vi "705_ProjectA.vi"() -> ()   [LabVIEW 2015]
uses:
  <vilib>/Utility/error.llb/DialogType.ctl
  <vilib>/Platform/TimedLoop/XDataNode/timing_clust.ctl
  <vilib>/Platform/TimedLoop/XDataNode/nitl_modes.ctl
  <vilib>/Platform/TimedLoop/XDataNode/wakeup.ctl
  <vilib>/DAQmx/read.llb/DAQmx Read (Digital Bool 1Line 1Point).vi
  <vilib>/DAQmx/read.llb/DAQmx Read (Counter DBL 1Chan 1Samp).vi
  <vilib>/DAQmx/write.llb/DAQmx Write (Analog DBL 1Chan 1Samp).vi
  <vilib>/DAQmx/read.llb/DAQmx Read (Analog 1D DBL NChan 1Samp).vi
  <vilib>/DAQmx/create/channels.llb/DAQmx Create Channel (AI-Voltage-Basic).vi
  <vilib>/DAQmx/create/channels.llb/DAQmx Create Channel (AO-Voltage-Basic).vi
  <vilib>/DAQmx/create/channels.llb/DAQmx Create Channel (CI-Count Edges).vi
  <vilib>/DAQmx/create/channels.llb/DAQmx Create Channel (DI-Digital Input).vi
  Global 1.vi
  <vilib>/DAQmx/miscellaneous.llb/DAQmx Fill In Error Info.vi
  <vilib>/Analysis/3filter.llb/Butterworth Filter (DBL).vi
  <vilib>/Platform/TimedLoop/XDataNode/XDataNode.xnode
  <vilib>/Platform/TimedLoop/XDataNode/XDNodeRunTimeDep.lvlib
  <vilib>/ptbypt/NI_PtbyPt.lvlib
  <vilib>/Analysis/NI_AALBase.lvlib
panel:
  in  "stop":bool
  out "Encoder":dbl
  out "position":dbl
  out "Current Position":dbl(graph)
  in  "RESET":bool
  out "timer":dbl
  out "Motor Speed":dbl[](graph)
  out "Current Draw":dbl(graph)
  out "DAQ O/P and Motor Voltage":cluster{dbl, "Applied Motor Voltage":dbl}(graph)
  out "Motor Position 2":dbl(graph)
  out "Motor Acceleration":dbl(graph)
  in  "Tab Control":T1(tab)
  in  "Physical Channel Current":tag="Dev5/ai0"
  in  "Physical Channel Tachometer":tag="Dev5/ai0"
  in  "Physical Channel Voltage":tag="Dev5/ai0"
  in  "max moter voltage":dbl
  in  "min moter voltage":dbl
  in  "Time Period (ms)":dbl
  in  "Motor Voltage Applied":dbl(slide) min=-5.0 max=5.0 step=0.1 scale=-5.0..5.0 scale format="%#.2g"
  out "element 2":bool
  out "Motor Position":dbl
  in  "counter":tag
  in  "Lines Port0/line6":tag
  in  "Start Moving":bool
  in  "Position between gripper":dbl
  out "Position":cluster{dbl, "Position between gripper":dbl}(graph)
  in  "pVoltage Range":cluster{"output high":dbl, "output low":dbl}={"output high"=100.0, "output low"=-100.0}
  in  "pPID gains":T2={"proportional gain (Kp)"=1.0, "integral gain (Ki)"=0.01, "derivative gain (Kd)"=0.0} {"derivative gain (Kd)" format="%.3f"; "integral gain (Ki)" format="%.3f"; "proportional gain (Kp)" format="%.3f"}
  in  "Start Gripping":bool
  in  "Desired Force":dbl
  out "Force":cluster{"Desired Force":dbl, dbl}(graph)
  in  "fVoltage Range":cluster{"output high":dbl, "output low":dbl}
  in  "fPID gains":T2={"proportional gain (Kp)"=1.0, "integral gain (Ki)"=0.01, "derivative gain (Kd)"=0.0} {"derivative gain (Kd)" format="%.3f"; "integral gain (Ki)" format="%.3f"; "proportional gain (Kp)" format="%.3f"}
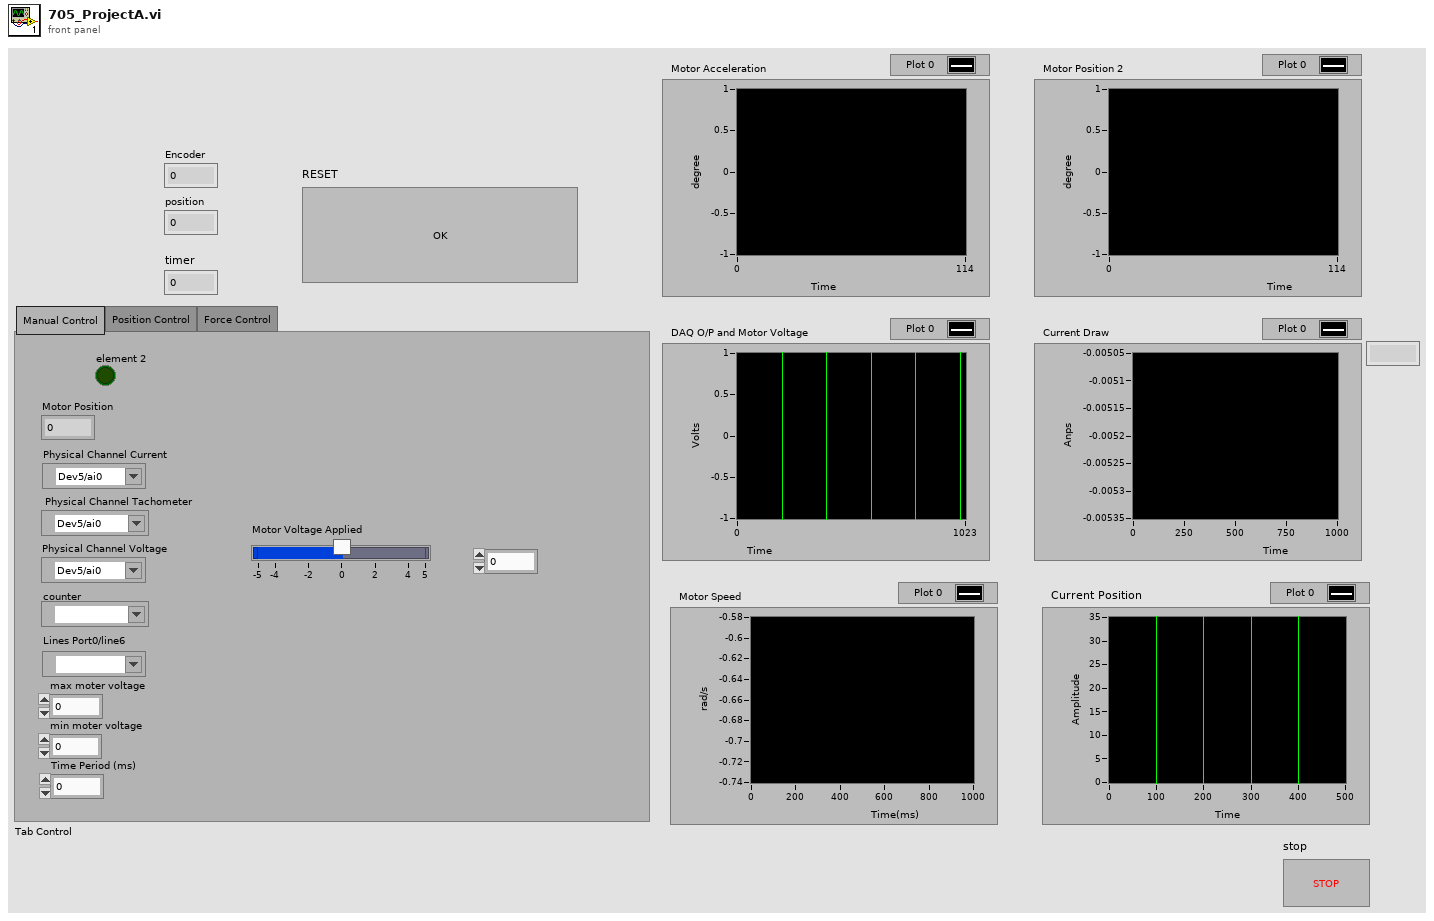
[diagram p1: front panel]
types:
  T1 = enum32{"Manual Control", "Position Control", "Force Control"}
  T2 = cluster{"proportional gain (Kp)":dbl, "integral gain (Ki)":dbl, "derivative gain (Kd)":dbl}
  T3 = typedef "DialogType.ctl" = u16
  T4 = typedef "XDNodeRunTimeDep.lvlib/timing_clust.ctl" = cluster{"Expected End [f-1]":u64, "Actual End [f-1]":u64, "Finished Late? [f-1]":bool, "Expected End [i-1]":u64, "Actual End [i-1]":u64, "Finished Late? [i-1]":bool, "Expected Start [i]":u64, "Actual Start [i]":u64, "Expected Start [f]":u64, "Actual Start [f]":u64, "Source Name":string, "Structure Name":string, "Period":i64, "Deadline":i64, "Offset":i64, "Start":i64, "Priority":i32, "Timeout":i32, "Mode":T5, "Wakeup Reason":T6, "Error":errorcluster, "Source Type":string, "Secondary Source Type":string, "Global End Time":u64, "Global Start Time":u64, "Frame Duration":u64, "Iteration Duration":u64, "Assigned CPU":i32, "I/O Scan Engine Mode":u32}
  T5 = typedef "XDNodeRunTimeDep.lvlib/nitl_modes.ctl" = enum32{"No Change", "Process missed periods, maintain original phase", "Discard missed periods, maintain original phase", "Process missed periods, ignore original phase", "Discard missed periods, ignore original phase"}
  T6 = typedef "XDNodeRunTimeDep.lvlib/wakeup.ctl" = enum32{"Normal", "Aborted", "Asynchronous wakeup", "Timing source error", "Timed loop error", "Timeout"}
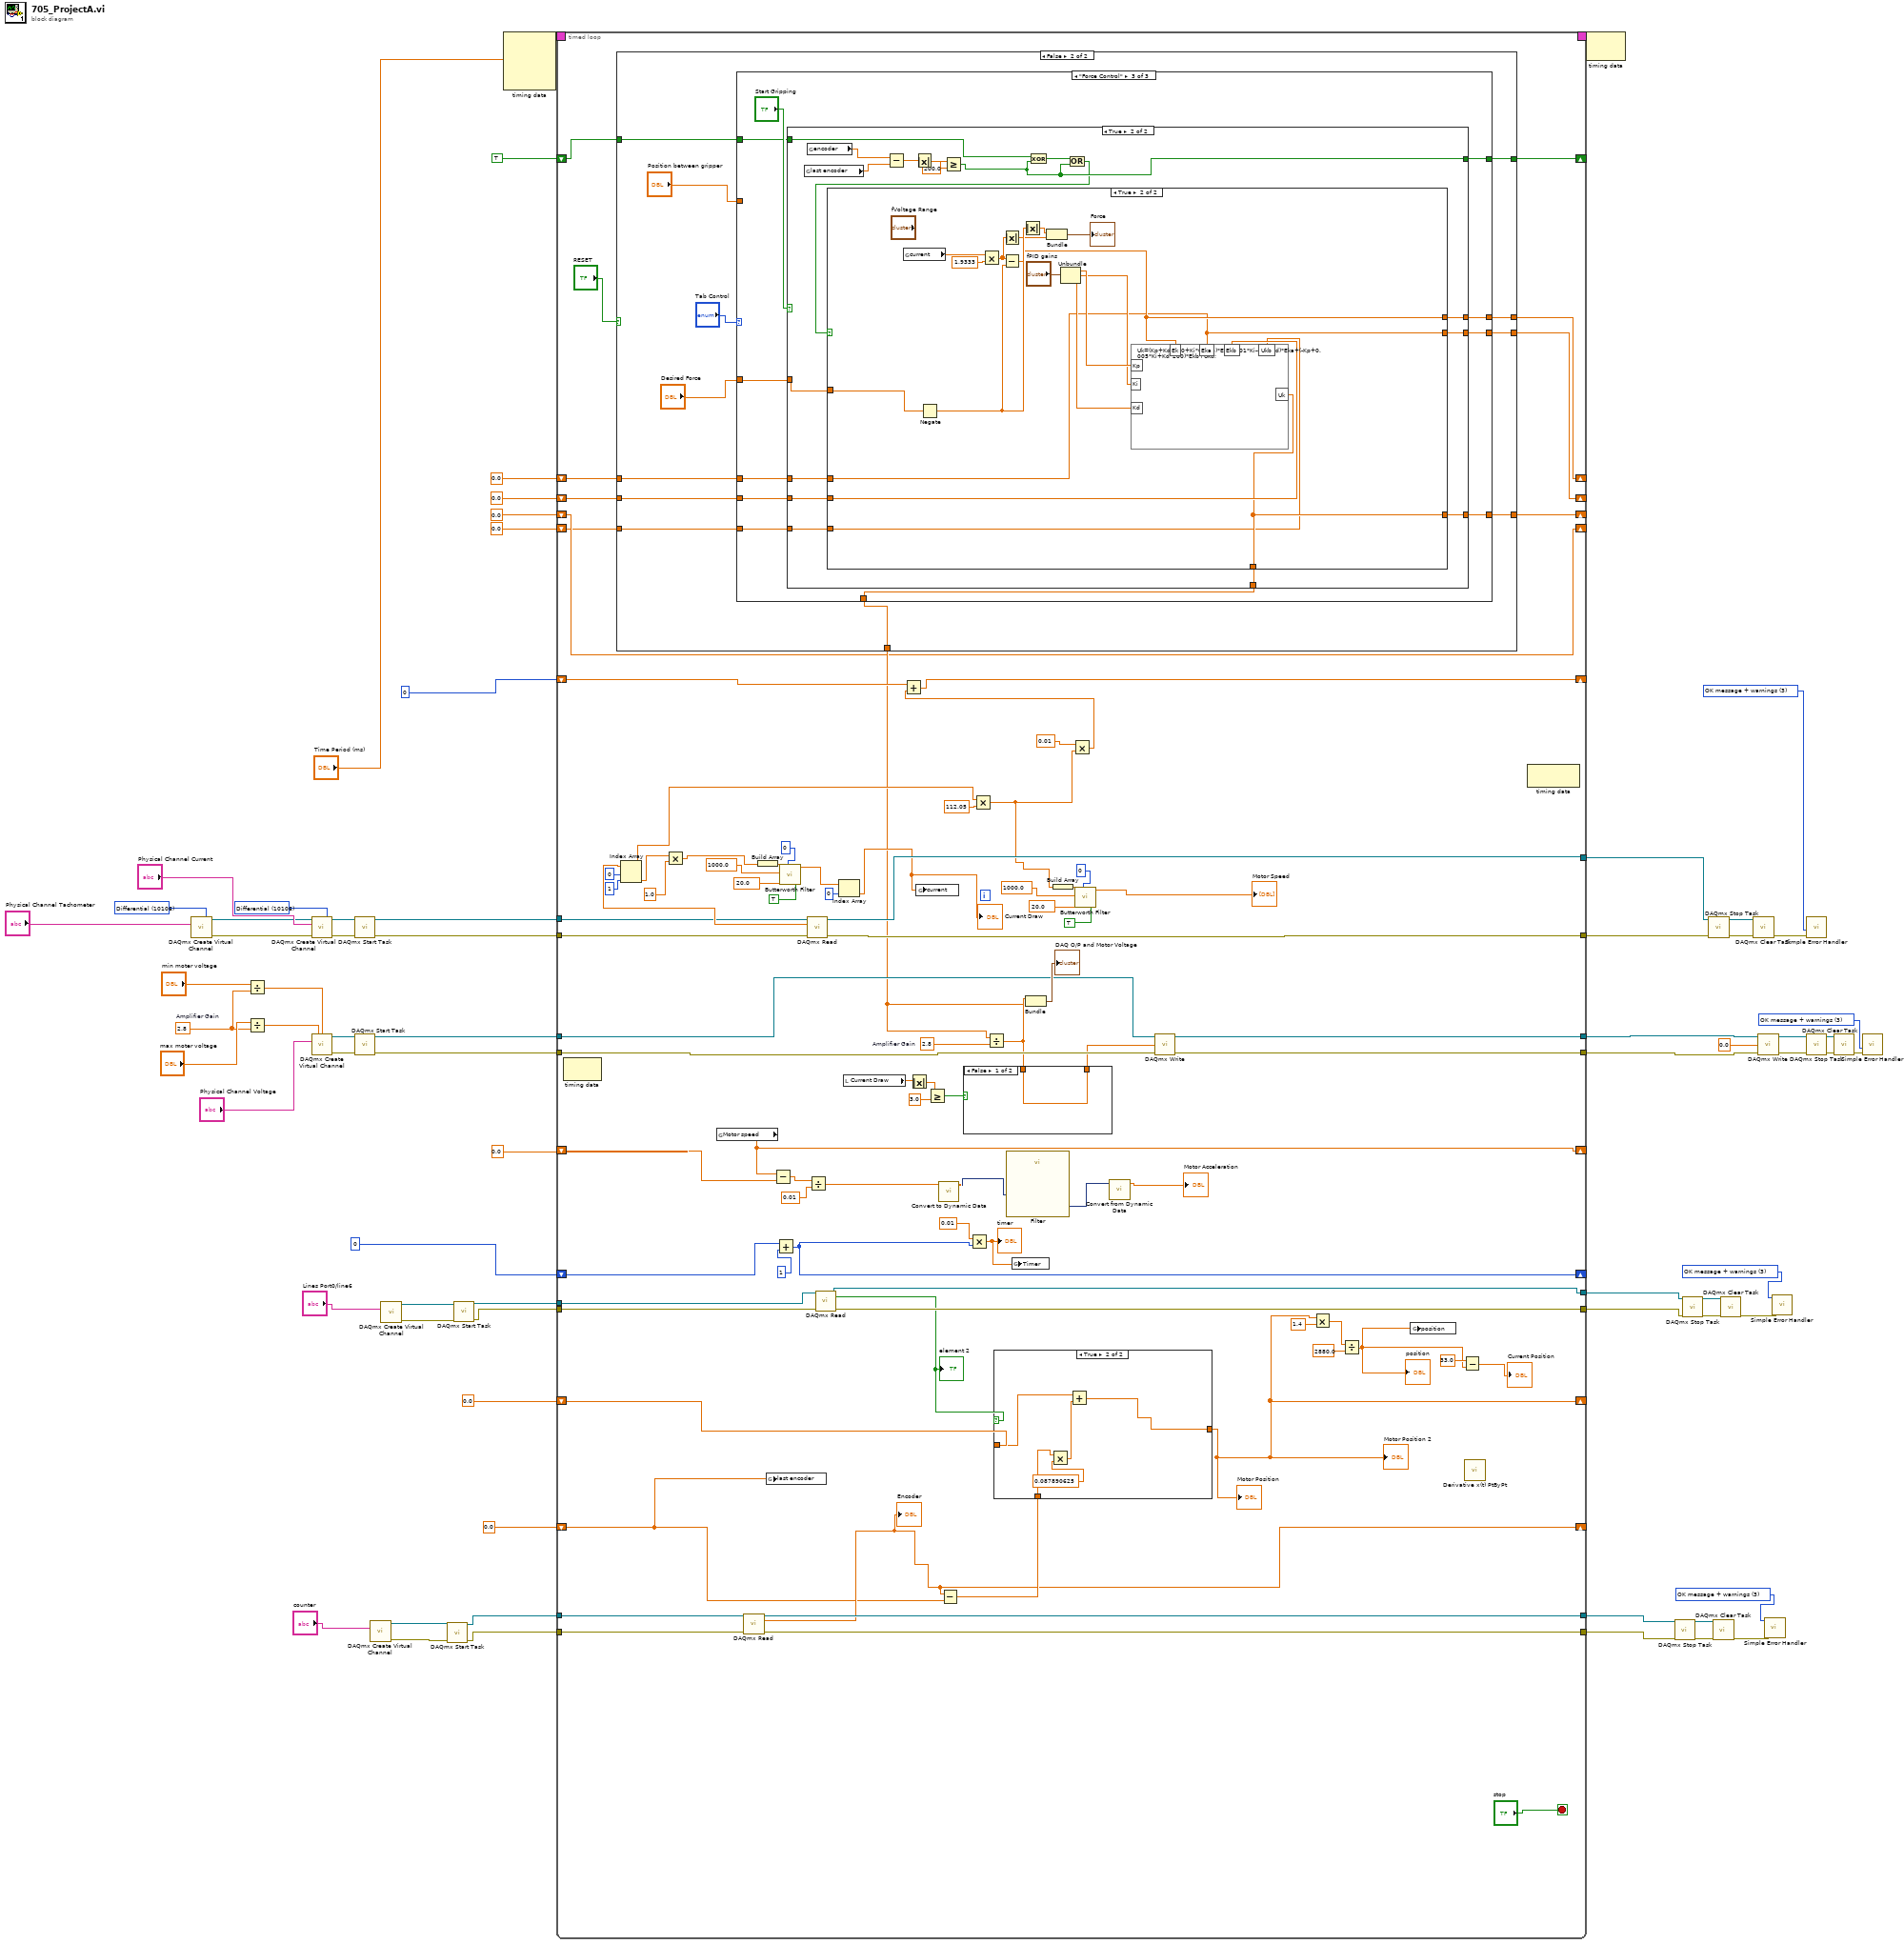
[diagram p0: block diagram]
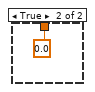
[diagram p2: hidden frame]
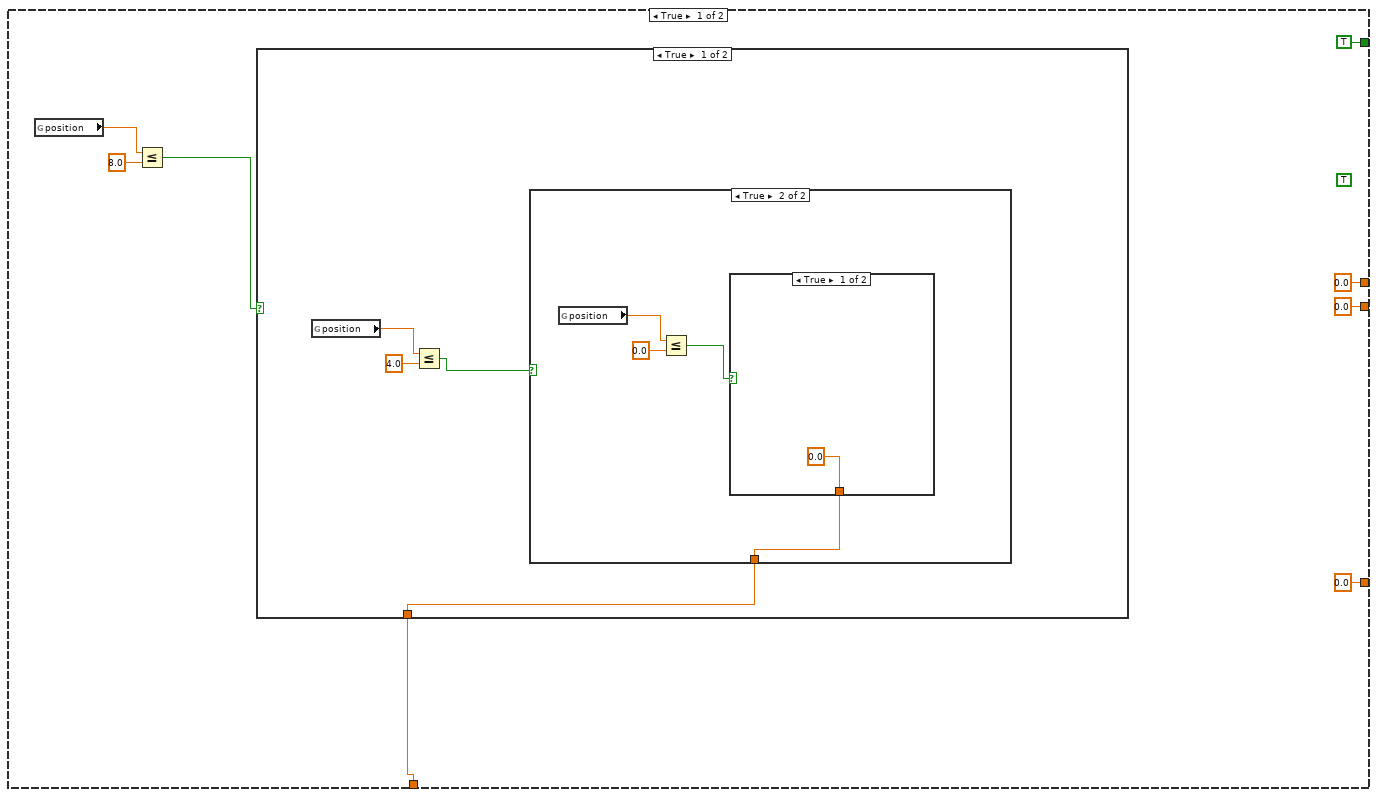
[diagram p3: hidden frame]
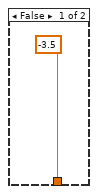
[diagram p4: hidden frame]
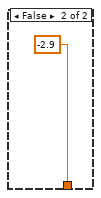
[diagram p5: hidden frame]
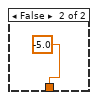
[diagram p6: hidden frame]
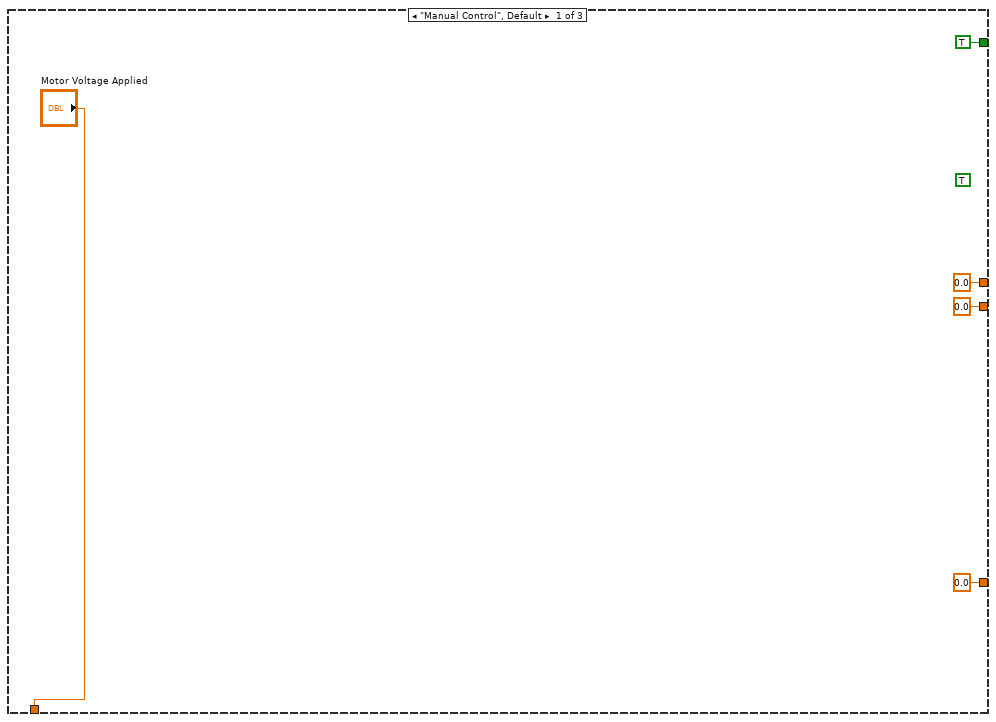
[diagram p7: hidden frame]
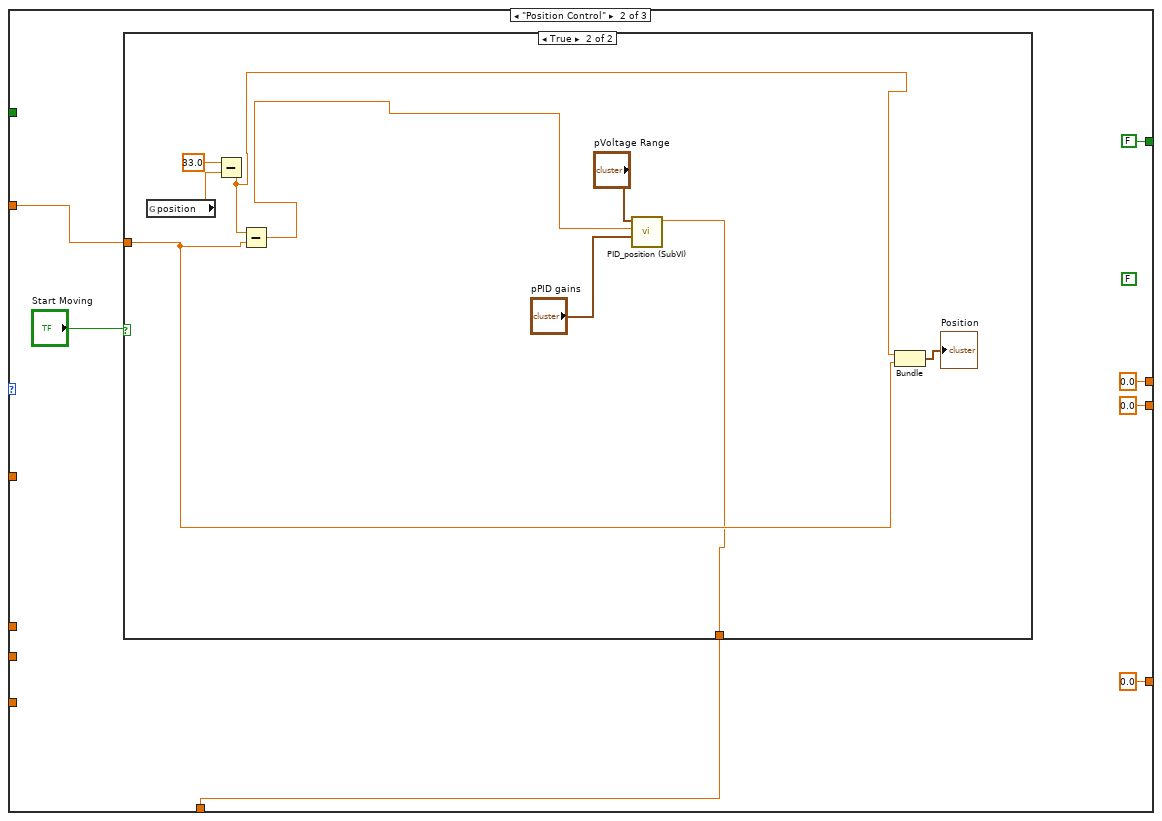
[diagram p8: hidden frame]
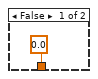
[diagram p9: hidden frame]
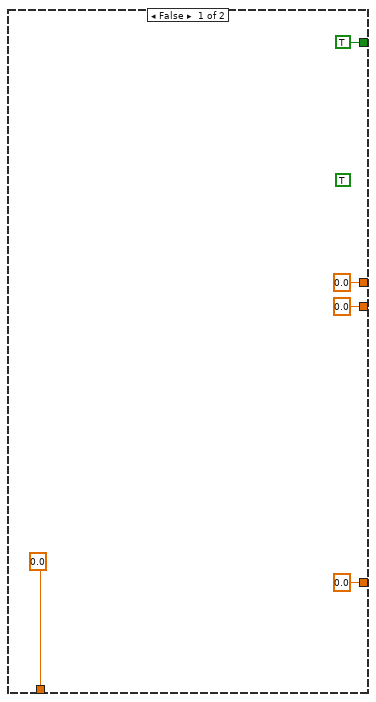
[diagram p10: hidden frame]
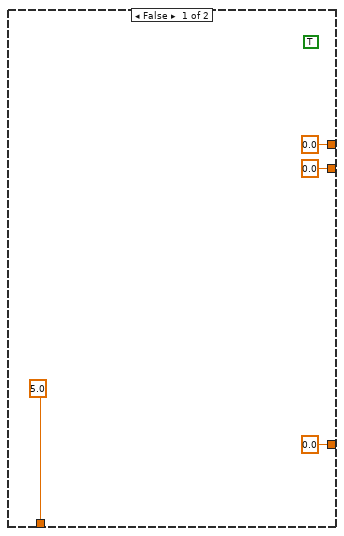
[diagram p11: hidden frame]
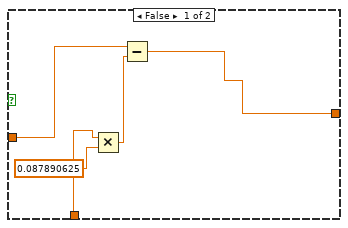
[diagram p12: hidden frame]
diagram:
  w12 = T3 3 items=["no dialog", "OK message", "continue or stop message", "OK message + warnings", "continue/stop + warnings"] ("type of dialog (OK msg:1)")
  w23 = T3 3 items=["no dialog", "OK message", "continue or stop message", "OK message + warnings", "continue/stop + warnings"] ("type of dialog (OK msg:1)")
  w33 = T3 3 items=["no dialog", "OK message", "continue or stop message", "OK message + warnings", "continue/stop + warnings"] ("type of dialog (OK msg:1)")
  w34 = T3 3 items=["no dialog", "OK message", "continue or stop message", "OK message + warnings", "continue/stop + warnings"] ("type of dialog (OK msg:1)")
  w58 = 2.8  # Amplifier Gain
  w60 = 10106 items=["default"=-1, "RSE"=10083, "NRSE"=10078, "Differential"=10106, "Pseudodifferential"=12529] ("input terminal configuration")
  w61 = 10106 items=["default"=-1, "RSE"=10083, "NRSE"=10078, "Differential"=10106, "Pseudodifferential"=12529] ("input terminal configuration")
  n1 = call-poly <vilib>:"DAQmx Create Virtual Channel.vi"("input terminal configuration"=w61, "physical channels"="Physical Channel Tachometer") -> ("task out"=w69:refnum<k21>, "error out"=w67:errorcluster)  [unwired: 12 in]
  n2 = Divide(x="min moter voltage", y=w58) -> (x/y=w56:dbl)
  n3 = Divide(x="max moter voltage", y=w58) -> (x/y=w57:dbl)
  n4 = call-poly <vilib>:"DAQmx Create Virtual Channel.vi"("task in"=w69, "input terminal configuration"=w60, "physical channels"="Physical Channel Current", "error in"=w67) -> ("task out"=w65:refnum<k21>, "error out"=w66:errorcluster)  [unwired: 10 in]
  n5 = call-poly <vilib>:"DAQmx Create Virtual Channel.vi"("maximum value"=w57, "minimum value"=w56, "physical channels"="Physical Channel Voltage") -> ("task out"=w63:refnum<k21>, "error out"=w62:errorcluster)  [unwired: 11 in]
  n6 = call <vilib>:"DAQmx Start Task.vi"("task/channels in"=w65, "error in"=w66) -> ("task out"=w52:refnum<k21>, "error out"=w51:errorcluster)  [unwired: 12 in]
  n7 = call <vilib>:"DAQmx Start Task.vi"("task/channels in"=w63, "error in"=w62) -> ("task out"=w50:refnum<k21>, "error out"=w49:errorcluster)  [unwired: 12 in]
  n8 = call-poly <vilib>:"DAQmx Create Virtual Channel.vi"("counter"="counter") -> ("task out"=w27:refnum<k21>, "error out"=w28:errorcluster)  [unwired: 13 in]
  n9 = call-poly <vilib>:"DAQmx Create Virtual Channel.vi"("lines"="Lines Port0/line6") -> ("task out"=w15:refnum<k21>, "error out"=w16:errorcluster)  [unwired: 13 in]
  n10 = call <vilib>:"DAQmx Start Task.vi"("task/channels in"=w27, "error in"=w28) -> ("task out"=w25:refnum<k21>, "error out"=w24:errorcluster)  [unwired: 12 in]
  n11 = call <vilib>:"DAQmx Start Task.vi"("task/channels in"=w15, "error in"=w16) -> ("task out"=w13:refnum<k21>, "error out"=w14:errorcluster)  [unwired: 12 in]
  n12 = node-c288("Time Period (ms)") -> (w54:T4)  [unwired: 3 in]
  n13 = timed-loop {
    timing: w54 -> [_]
    timing-out: [_] -> w53
    tunnel: w52 -> [w134]
    tunnel: w51 -> [w149]
    tunnel: w50 -> [w148]
    tunnel: w49 -> [w147]
    tunnel: [w152] -> w42
    tunnel: [w151] -> w41
    tunnel: [w138] -> w46
    tunnel: [w150] -> w47
    shift-right: [w144] -> _
    shift-left: 0 -> [w145]
    shift-right: [w137] -> _
    shift-left: 0 -> [w142]
    shift-right: [w116] -> _
    shift-left: 0.0 ("data") -> [w79]
    shift-right: [w130] -> _
    shift-left: 0.0 -> [w135]
    shift-right: [w126] -> _
    shift-left: 0.0 -> [w129]
    tunnel: w25 -> [w120]
    tunnel: w24 -> [w119]
    tunnel: [w118] -> w20
    tunnel: [w117] -> w19
    tunnel: w14 -> [w115]
    tunnel: w13 -> [w114]
    tunnel: [w113] -> w8
    tunnel: [w112] -> w7
    shift-right: [w83] -> _
    shift-left: TRUE -> [w82]
    shift-right: [w77] -> _
    shift-left: 0.0 -> [w76]
    shift-right: [w75] -> _
    shift-left: 0.0 -> [w74]
    shift-right: [w73] -> _
    shift-left: 0.0 ("Uk") -> [w72]
    shift-right: [w72] -> _
    shift-left: 0.0 ("Uk") -> [w71]
    stop <- "stop" stop-if-true
    w158 = 2.8  # Amplifier Gain
    n14 = node-c288() -> ()  [unwired: 1 in, 1 out]
    n15 = case shown="False" "RESET" {
      tunnel: [w165 w191] -> w78
      tunnel: [TRUE w188] -> w83
      tunnel: w82 -> [_ w187]
      tunnel: [0.0 w186] -> w77
      tunnel: w76 -> [_ w185]
      tunnel: [0.0 w184] -> w75
      tunnel: w74 -> [_ w183]
      tunnel: [0.0 ("Uk") w182] -> w73
      tunnel: w71 -> [_ w181]
      frame True {
        (unwired) TRUE
        n16 = global read "Global 1.vi" "position"() -> (w167:dbl)
        n17 = Less Or Equal?(x=w167, y=8.0) -> (x <= y?=w166:bool)
        n18 = case shown="True" w166 {
          tunnel: [w169 -5.0] -> w165
          frame True {
            n19 = global read "Global 1.vi" "position"() -> (w171:dbl)
            n20 = Less Or Equal?(x=w171, y=4.0) -> (x <= y?=w170:bool)
            n21 = case shown="True" w170 {
              tunnel: [-3.5 w174] -> w169
              frame False {
              }
              frame True {
                n22 = global read "Global 1.vi" "position"() -> (w176:dbl)
                n23 = Less Or Equal?(x=w176, y=0.0) -> (x <= y?=w175:bool)
                n24 = case shown="True" w175 {
                  tunnel: [0.0 -2.9] -> w174
                  frame True {
                  }
                  frame False {
                  }
                }
              }
            }
          }
          frame False {
          }
        }
      }
      frame False {
        n25 = case shown="\"Force Control\"" "Tab Control" {
          tunnel: ["Motor Voltage Applied" w203 w223] -> w191
          tunnel: "Position between gripper" -> [_ w204 _]
          tunnel: "Desired Force" -> [_ _ w224]
          tunnel: [TRUE FALSE w222] -> w188
          tunnel: w187 -> [_ _ w221]
          tunnel: [0.0 0.0 w220] -> w186
          tunnel: w185 -> [_ _ w219]
          tunnel: [0.0 0.0 w218] -> w184
          tunnel: w183 -> [_ _ w217]
          tunnel: [0.0 ("Uk") 0.0 ("Uk") w216] -> w182
          tunnel: w181 -> [_ _ w215]
          frame "Manual Control", Default {
            (unwired) TRUE
          }
          frame "Position Control" {
            (unwired) FALSE
            n26 = case shown="True" "Start Moving" {
              tunnel: w204 -> [_ w210]
              tunnel: [0.0 ("Vout") w207] -> w203
              frame False {
              }
              frame True {
                n27 = global read "Global 1.vi" "position"() -> (w213:dbl)
                n28 = Subtract(x=33.0, y=w213) -> (x-y=w211:dbl)
                n29 = Subtract(x=w211, y=w210) -> (x-y=w209:dbl)
                n30 = call "PID_position (SubVI).vi"("PID gains in"="pPID gains", "setpoint"=w209, "Voltage Range in"="pVoltage Range") -> ("Vout"=w207:dbl)  [unwired: 8 in]
                n31 = Bundle(w211, "Position between gripper"=w210) -> (→"Position":cluster{dbl, "Position between gripper":dbl})  [unwired: 1 in]
              }
            }
          }
          frame "Force Control" {
            n32 = case shown="True" "Start Gripping" {
              tunnel: w224 -> [_ w246]
              tunnel: [0.0 ("Vout") w247] -> w223
              tunnel: [TRUE w239] -> w222
              tunnel: w221 -> [_ w240]
              tunnel: [0.0 w236] -> w220
              tunnel: w219 -> [_ w235]
              tunnel: [0.0 w234] -> w218
              tunnel: w217 -> [_ w233]
              tunnel: [0.0 ("Uk") w232] -> w216
              tunnel: w215 -> [_ w231]
              frame False {
                (unwired) TRUE
              }
              frame True {
                n33 = global read "Global 1.vi" "last encoder"() -> (w244:dbl)
                n34 = global read "Global 1.vi" "encoder"() -> (w245:dbl)
                n35 = Subtract(x=w245, y=w244) -> (x-y=w243:dbl)
                n36 = Absolute Value(x=w243) -> (abs(x)=w242:dbl)
                n37 = Greater Or Equal?(x=w242, y=200.0) -> (x >= y?=w239:bool)
                n38 = Exclusive Or(1:w239, 2:w240) -> (0:w238:bool)
                n39 = Or(x=w238, y=w239) -> (x .or. y?=w237:bool)
                n40 = case shown="True" w237 {
                  tunnel: [5.0 w253] -> w247
                  tunnel: w246 -> [_ w268]
                  tunnel: [0.0 w256] -> w236
                  tunnel: w235 -> [_ w255]
                  tunnel: [0.0 w255] -> w234
                  tunnel: w233 -> [_ w254]
                  tunnel: [0.0 ("Uk") w253] -> w232
                  tunnel: w231 -> [_ w252]
                  frame False {
                    (unwired) TRUE
                  }
                  frame True {
                    n41 = global read "Global 1.vi" "current"() -> (w264:dbl)
                    n42 = Negate(x=w268) -> (-x=w263:dbl)
                    n43 = Multiply(x=w264, y=1.9333) -> (x*y=w265:dbl)
                    n44 = Absolute Value(x=w265) -> (abs(x)=w262:dbl)
                    n45 = Subtract(x=w265, y=w263) -> (x-y=w256:dbl)
                    n46 = Absolute Value(x=w263) -> (abs(x)=w261:dbl)
                    n47 = Bundle(w261, w262) -> (→"Force":cluster{dbl, dbl})  [unwired: 1 in]
                    n48 = Unbundle("fPID gains") -> ("proportional gain (Kp)"=w259:dbl, "integral gain (Ki)"=w258:dbl, "derivative gain (Kd)"=w257:dbl)
                    n49 = formula code="Uk=(Kp+Kd*200+Ki*0.005)*Ek+(0.01*Ki-400*Kd)*Eka+(-Kp+0.005*Ki+Kd*200)*Ekb+Ukb;"("Kp"=w259, "Ki"=w258, "Kd"=w257, "Ek"=w256, "Eka"=w255, "Ekb"=w254, "Ukb"=w252) -> ("Uk"=w253:dbl)
                  }
                }
              }
            }
          }
        }
      }
    }
    n50 = global read "Global 1.vi" "Motor speed"() -> (w126:dbl)
    n51 = call-poly <vilib>:"DAQmx Read.vi"("task/channels in"=w120, "error in"=w119) -> ("task out"=w117:refnum<k21>, "data"=w116:dbl, "error out"=w118:errorcluster)  [unwired: 11 in]
    "Encoder" <- w116
    n52 = global write "Global 1.vi" "last encoder"(w79) -> ()
    n53 = Subtract(x=w126, y=w129) -> (x-y=w128:dbl)
    n54 = Add(x=w145, y=1) -> (x+y=w144:i32)
    n55 = call-poly <vilib>:"DAQmx Read.vi"("task/channels in"=w134, "error in"=w149) -> ("task out"=w150:refnum<k21>, "data"=w139:dbl[], "error out"=w138:errorcluster)  [unwired: 11 in]
    n56 = Index Array(array=w139, index #1=0, index #2=1) -> (element #1=w109:dbl, element #2=w110:dbl)
    n57 = Multiply(x=w110, y=1.0) -> (x*y=w87:dbl)
    n58 = Build Array(w87) -> (w89:dbl[])
    n59 = call-poly <vilib>:"Butterworth Filter.vi"("init/cont (init:F)"=TRUE, "filter type"=0 ("index"), "low cutoff freq: fl"=20.0, "sampling freq: fs"=1000.0, "X"=w89) -> ("Filtered X"=w86:dbl[])  [unwired: 3 in, 1 out]
    n60 = Divide(x=w128, y=0.01) -> (x/y=w125:dbl)
    n61 = call-poly <vilib>:"DAQmx Read.vi"("task/channels in"=w114, "error in"=w115) -> ("task out"=w112:refnum<k21>, "data"=w111:bool, "error out"=w113:errorcluster)  [unwired: 11 in]
    "element 2" <- w111
    n62 = Index Array(array=w86, index=0) -> (element=w84:dbl)
    "Current Draw" <- w84
    n63 = local read "Current Draw"() -> (w98:dbl)
    n64 = Absolute Value(x=w98) -> (abs(x)=w97:dbl)
    n65 = global write "Global 1.vi" "current"(w84) -> ()
    n66 = Greater Or Equal?(x=w97, y=3.0) -> (x >= y?=w95:bool)
    n67 = call "Convert to Dynamic Data"("Double"=w125) -> ("Dynamic Data Type"=w123:dynamicdata)  [unwired: 3 in]
    n68 = Subtract(x=w116, y=w79) -> (x-y=w136:dbl)
    n69 = Multiply(x=0.01, y=w144) -> (x*y=w121:dbl)
    "timer" <- w121
    n70 = Multiply(x=w109, y=112.05) -> (x*y=w104:dbl)
    n71 = Divide(x=w78, y=w158) -> (x/y=w81:dbl)
    n72 = case shown="False" w95 {
      tunnel: [w159 0.0] -> w94
      tunnel: w81 -> [w159 _]
      frame False {
      }
      frame True {
      }
    }
    n73 = case shown="True" w111 {
      tunnel: w136 -> [w270 w278]
      tunnel: w135 -> [w271 w275]
      tunnel: [w269 w276] -> w130
      frame False {
        n74 = Multiply(x=w270, y=0.087890625) -> (x*y=w272:dbl)
        n75 = Subtract(x=w271, y=w272) -> (x-y=w269:dbl)
      }
      frame True {
        n76 = Multiply(x=w278, y=0.087890625) -> (x*y=w277:dbl)
        n77 = Add(x=w275, y=w277) -> (x+y=w276:dbl)
      }
    }
    "Motor Position 2" <- w130
    "Motor Position" <- w130
    n78 = call "Filter"("Signal"=w123) -> ("Filtered Signal"=w122:dynamicdata)  [unwired: 9 in, 1 out]
    n79 = global write "Global 1.vi" "Timer"(w121) -> ()
    n80 = Bundle(w81, "Uk"=w78) -> (→"DAQ O/P and Motor Voltage":cluster{dbl, "Uk":dbl})  [unwired: 1 in]
    n81 = Build Array(w104) -> (w105:dbl[])
    n82 = Multiply(x=0.01, y=w104) -> (x*y=w141:dbl)
    n83 = Add(x=w142, y=w141) -> (x+y=w137:dbl)
    n84 = call-poly <vilib>:"Butterworth Filter.vi"("init/cont (init:F)"=TRUE, "filter type"=0 ("index"), "low cutoff freq: fl"=20.0, "sampling freq: fs"=1000.0, "X"=w105) -> ("Filtered X"=→"Motor Speed":dbl[])  [unwired: 3 in, 1 out]
    n85 = call "Convert from Dynamic Data"("Dynamic Data Type"=w122) -> ("Scalar"=→"Motor Acceleration":dbl)  [unwired: 3 in]
    n86 = call-poly <vilib>:"DAQmx Write.vi"("task/channels in"=w148, "data"=w94, "error in"=w147) -> ("task out"=w152:refnum<k21>, "error out"=w151:errorcluster)  [unwired: 10 in, 1 out]
    n87 = Multiply(x=w130, y=1.4) -> (x*y=w131:dbl)
    n88 = Divide(x=w131, y=2880.0) -> (x/y=w100:dbl)
    "position" <- w100
    n89 = global write "Global 1.vi" "position"(w100) -> ()
    n90 = Subtract(x=33.0, y=w100) -> (x-y=→"Current Position":dbl)
    n91 = call <vilib>:"Derivative x(t) PtByPt.vi"() -> ()  [unwired: 4 in, 2 out]
    n92 = node-c288() -> ()  [unwired: 1 in, 1 out]
  }
  n93 = node-c288(w53) -> ()  [unwired: 1 out]
  n94 = call <vilib>:"DAQmx Stop Task.vi"("task/channels in"=w19, "error in"=w20) -> ("task out"=w18:refnum<k21>, "error out"=w21:errorcluster)  [unwired: 12 in]
  n95 = call <vilib>:"DAQmx Stop Task.vi"("task/channels in"=w7, "error in"=w8) -> ("task out"=w9:refnum<k21>, "error out"=w10:errorcluster)  [unwired: 12 in]
  n96 = call <vilib>:"DAQmx Stop Task.vi"("task/channels in"=w47, "error in"=w46) -> ("task out"=w44:refnum<k21>, "error out"=w45:errorcluster)  [unwired: 12 in]
  n97 = call <vilib>:"DAQmx Clear Task.vi"("task in"=w18, "error in"=w21) -> ("error out"=w22:errorcluster)  [unwired: 13 in]
  n98 = call <vilib>:"DAQmx Clear Task.vi"("task in"=w9, "error in"=w10) -> ("error out"=w11:errorcluster)  [unwired: 13 in]
  n99 = call <vilib>:"DAQmx Clear Task.vi"("task in"=w44, "error in"=w45) -> ("error out"=w43:errorcluster)  [unwired: 13 in]
  n100 = call-poly <vilib>:"DAQmx Write.vi"("task/channels in"=w42, "data"=0.0, "error in"=w41) -> ("task out"=w35:refnum<k21>, "error out"=w36:errorcluster)  [unwired: 10 in, 1 out]
  n101 = call <vilib>:"Simple Error Handler.vi"("error code (no error:0)"=w23, "error in (no error)"=w22) -> ()  [unwired: 3 in, 5 out]
  n102 = call <vilib>:"Simple Error Handler.vi"("error code (no error:0)"=w12, "error in (no error)"=w11) -> ()  [unwired: 3 in, 5 out]
  n103 = call <vilib>:"Simple Error Handler.vi"("type of dialog (OK msg:1)"=w34, "error in (no error)"=w43) -> ()  [unwired: 3 in, 5 out]
  n104 = call <vilib>:"DAQmx Stop Task.vi"("task/channels in"=w35, "error in"=w36) -> ("task out"=w38:refnum<k21>, "error out"=w39:errorcluster)  [unwired: 12 in]
  n105 = call <vilib>:"DAQmx Clear Task.vi"("task in"=w38, "error in"=w39) -> ("error out"=w37:errorcluster)  [unwired: 13 in]
  n106 = call <vilib>:"Simple Error Handler.vi"("type of dialog (OK msg:1)"=w33, "error in (no error)"=w37) -> ()  [unwired: 3 in, 5 out]
